vi "USRP Dummy DMA (Host).vi"() -> ()   [LabVIEW 2016]
uses:
  <vilib>/userdefined/High Color/nirio_resource_hc.ctl
  <vilib>/FPGAPlugInAG/USRP 294xR; 295xR 200 MSps/niLvFpga_Open_USRP 294xR; 295xR 200 MSps.vi
  <vilib>/rvi/interface/common/dynamic/niFpgaDynamicAddResources.vi
  <vilib>/Utility/error.llb/Error Cluster From Error Code.vi
  <vilib>/rvi/errors/niLvFpgaAdjustHostInterfaceError.vi
  <vilib>/rvi/interface/common/niFpgaWaitOnOcc.vi
  <vilib>/FPGAPlugInAG/Dynamic/niLvFpga_Close_Dynamic.vi
  <vilib>/rvi/interface/nirviOpenFPGA/nirviOpenFPGA.xnode
  FPGA Bitfiles/USRP-RIO-Streami_DummyDMA_USRPDummy(FPGA)_-Xglc-1l0hs.lvbitx
  <vilib>/rvi/interface/nirviReadWriteControl/nirviReadWriteControl.xnode
  <vilib>/rvi/interface/nirviMethod/nirviMethod.xnode
  <vilib>/rvi/interface/nirviCloseFPGA/nirviCloseFPGA.xnode
  <vilib>/rvi/errors/niLvFpgaMergeErrorWithErrorCode.vi
  <vilib>/rvi/interface/Simulation/niFpgaSimulationCallBeginRW.vi
  <instrlib>/niUsrpRio/Config/v1/Host/niUsrpRio Config v1 Host.lvlib
  NiFpgaLv.dll
  <instrlib>/_niInstr/Basic Elements/v1/FPGA/niInstr Basic Elements v1 FPGA.lvlib
  <vilib>/FPGAPlugInAG/Dynamic/niLvFpga_StopFifo_Dynamic.vi
  <vilib>/FPGAPlugInAG/Dynamic/niLvFpga_ConfigureFifo_Dynamic.vi
  <vilib>/FPGAPlugInAG/Dynamic/niLvFpga_StartFifo_Dynamic.vi
  <vilib>/FPGAPlugInAG/Dynamic/niLvFpga_ReadFifo_Dynamic.vi
panel:
  out "FPGA Side FIFO":cluster{u32, u32}(slide) scale=0.0..1.0
  out "Host Side FIFO":cluster{u32, u32}(slide) scale=0.0..4294967295.0
  out "Data Loop":i32
  out "Fetch Loop":i32
  out "Control Loop":i32
  out "Host Transfer Count":u64
  in  "Number of Samples":u64=1024
  out "FPGA Transfer Count":u64
  in  "Send Data?":bool
  in  "stop":bool
  out "Elements Remaining":u32
  out "Data":u64[](array[numeric]) format="%.0x"
  out "Total Timeouts":u64
  out "Sticky Timeouts?":bool
  in  "Reset Total Timeouts?":bool
  out "Actual Depth":u32
  in  "Requested Depth":u32=1048576
  out "error out":errorcluster
  in  "error in (no error)":errorcluster
  in  "resource name":T1="PXI2Slot18Port1Dev1"
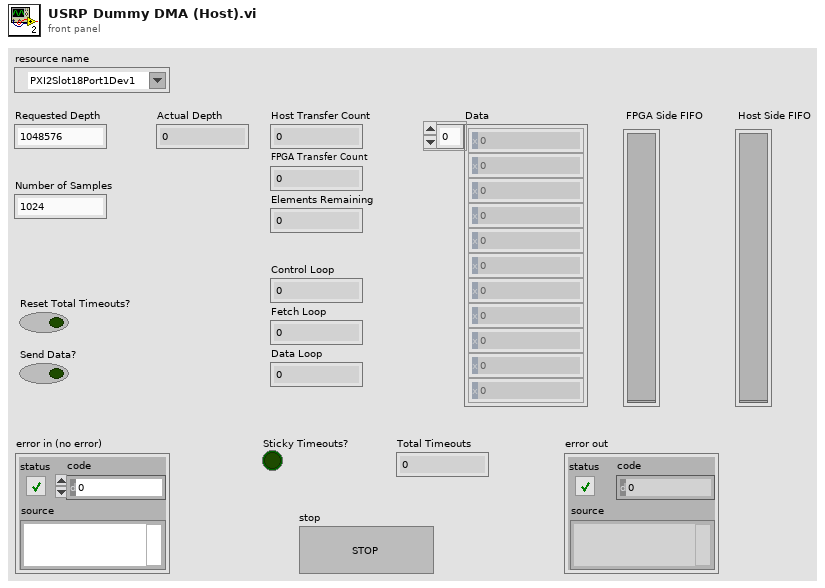
[diagram p1: front panel]
types:
  T1 = typedef "nirio_resource_hc.ctl" = tag
  T2 = typedef "niUsrpRio Config v1 Host.lvlib/niUsrpRio Session.ctl" = cluster{"FPGA Interface":refnum<k20>, "RIO Interface Number":u32, "Data Clock Rate":u32, "FPGA Data Clock Rate":u32, "Global Settings Register Bus":T3, "Radio 0 Settings Register Bus":T3, "Radio 1 Settings Register Bus":T3, "Radio Settings Bus Semaphore":T4, "DB Queues":T5[], "Characterization Data Valid?":bool, "EEPROM Header":T6, "Device Data Header":T7, "EEPROM Characterization Header":T8, "Characterization Data":T9[], "FPGA Current Version":u32, "FPGA Oldest Compatible Version":u32, "Fixed Logic Current Version":u32, "Fixed Logic Oldest Compatible Version":u32, "FPGA Radio Settings Bus Current Version":u32, "FPGA Radio Settings Bus Oldest Compatible Version":u32, "FPGA Board Config Current Version":u32, "FPGA Board Config Oldest Compatible Version":u32, "Daughterboard Clock Rate":u32, "daughterboard configuration session handles":u64[]}
  T3 = typedef "niInstr Register Bus v0 Host.lvlib/Register Bus Session.ctl" = refnum<queue>
  T4 = typedef "Semaphore RefNum" = refnum<k1>
  T5 = typedef "niUsrpRio Config v1 Host.lvlib/DB Queue Reference.ctl" = refnum<queue>
  T6 = typedef "niUsrpRio Config v1 Host.lvlib/EEPROM Header.ctl" = cluster{"Checksum":u32, "Product Code":u16, "Hardware Current Version":u16, "Hardware Oldest Compatible Version":u16, "EEPROM Map Current Version":u16, "EEPROM Map Oldest Compatible Version":u16, "User Password":string, "Pointer to Factory Header":u32, "Pointer to User Header":u32, "Recommended Interval":u16, "Number of Reserved Bytes":i32, "Number of Daughterboards":u8, "Daughterboard IDs":u16[], "Daughterboard Serial Numbers":string[]}
  T7 = typedef "niUsrpRio Config v1 Host.lvlib/EEPROM Device Data Header.ctl" = cluster{"Checksum":u32, "Number of Channels":u8, "Number of Gain Settings":u16[], "Pointer to Characterization Data":u32[], "Number of Reserved Bytes":i32, "Number of Frequencies":u16[]}
  T8 = typedef "niUsrpRio Config v1 Host.lvlib/EEPROM Characterization Header.ctl" = cluster{"Checksum":u32, "Date":timestamp, "Temperature":sgl, "Misc. Info":string, "Pointer to Device Data Header":u32, "Number of Reserved Bytes":i32}
  T9 = typedef "niUsrpRio Config v1 Host.lvlib/Characterization Data.ctl" = cluster{"Gains[dB]":dbl[], "Frequencies [Hz]":dbl[], "IQ Imbalance Table":T10[], "Measured Gains[dB]":dbl[][]}
  T10 = typedef "niUsrpRio Config v1 Host.lvlib/IQ Imbalance.ctl" = cluster{"Gain Imbalance [linear]":dbl, "Phase Imbalance [radians]":dbl, "Offset":cdb}
  T11 = cluster{"Current Amount Used":u32, "Maximum Amount Used":u32}
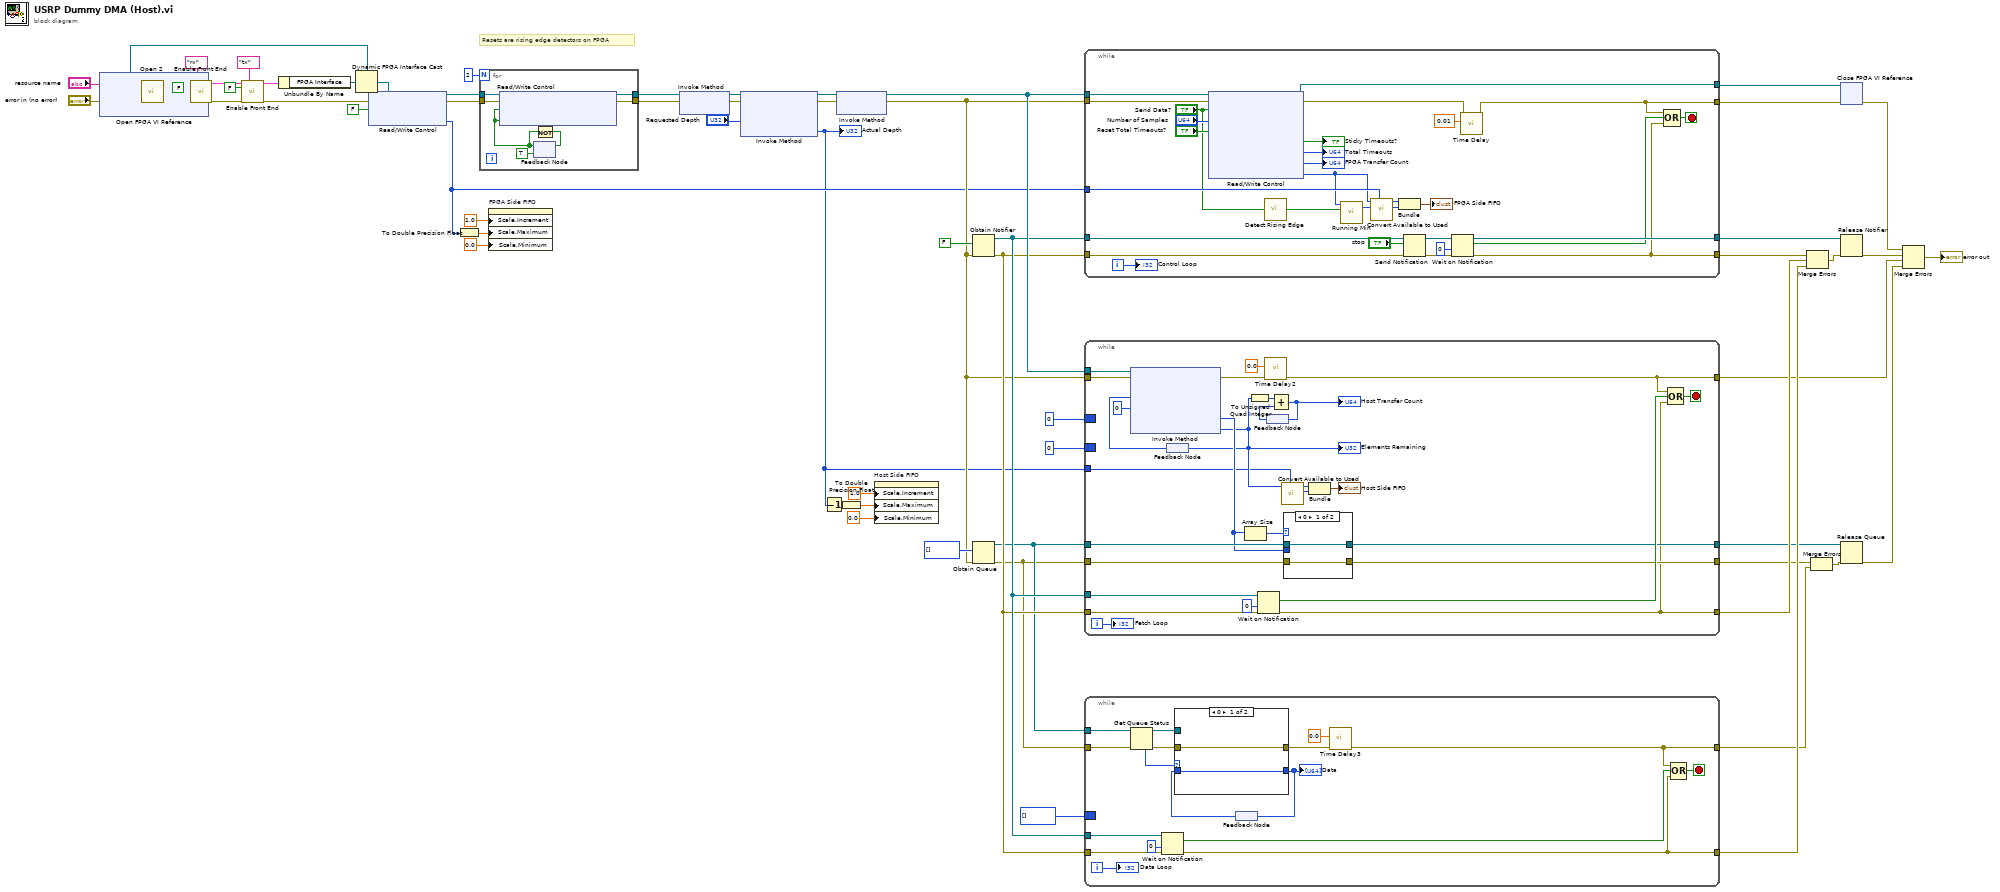
[diagram p0: block diagram]
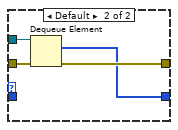
[diagram p2: hidden frame]
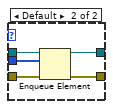
[diagram p3: hidden frame]
diagram:
  # "Resets are rising edge detectors on FPGA"
  n1 = xnode "Open FPGA VI Reference"("error in"="error in (no error)", "resource name"="resource name") -> ("FPGA VI Reference Out"=w42:refnum<k20>, "error out"=w43:errorcluster)
  n2 = call <instrlib>:"Open 2.vi"("fpga ref"=w42, "error in"=w43) -> ("niUsrpRio Session (out)"=w52:T2, "error out"=w57:errorcluster)  [unwired: 12 in]
  n3 = call <instrlib>:"Enable Front End.vi"("niUsrpRio Session"=w52, "scope"="rx", "enable"=FALSE, "error in"=w57) -> ("niUsrpRio Session (out)"=w53:T2, "error out"=w56:errorcluster)  [unwired: 10 in]
  n4 = call <instrlib>:"Enable Front End.vi"("niUsrpRio Session"=w53, "scope"="tx", "enable"=FALSE, "error in"=w56) -> ("niUsrpRio Session (out)"=w49:T2, "error out"=w48:errorcluster)  [unwired: 10 in]
  n5 = Unbundle By Name(w49) -> ("FPGA Interface"=w47:refnum<k20>)
  n6 = Dynamic FPGA Interface Cast(Session In=w42, Type=w47) -> (Session Out=w46:refnum<k20>)
  n7 = xnode "Read/Write Control"("FPGA VI Reference In"=w46, "error in"=w48, "Send Data?"=FALSE ("send data?")) -> ("FPGA VI Reference Out"=w19:refnum<k20>, "error out"=w18:errorcluster, "FPGA FIFO Depth"=w2:u32)
  n8 = To Double Precision Float(number=w2) -> (double precision float=w4:dbl)
  n9 = for {
    N: 2 -> [_]
    tunnel: w19 -> [w70]
    tunnel: w18 -> [w69]
    tunnel: [w68] -> w17
    tunnel: [w67] -> w16
    n10 = feedback #1(TRUE) -> (w65:bool)
    n11 = xnode "Read/Write Control"("FPGA VI Reference In"=w70, "error in"=w69, "Reset Total Timeouts?"=w65, "Reset FPGA Transfer Count?"=w65) -> ("FPGA VI Reference Out"=w68:refnum<k20>, "error out"=w67:errorcluster)
    n12 = Not(x=w65) -> (.not. x?=w64:bool)
    n13 = feedback-in #1(w64) -> ()
  }
  n14 = property on="FPGA Side FIFO" class="Slide (strict)"("Scale.Increment"=1.0 ("Scale.Range:Increment"), "Scale.Maximum"=w4, "Scale.Minimum"=0.0 ("Scale.Range:Minimum")) -> ()  [unwired: 2 in, 2 out]
  n15 = xnode "Invoke Method"("FPGA VI Reference In"=w17, "error in"=w16) -> ("FPGA VI Reference Out"=w63:refnum<k20>, "error out"=w62:errorcluster)
  n16 = xnode "Invoke Method"("FPGA VI Reference In"=w63, "error in"=w62, "Requested Depth"="Requested Depth") -> ("FPGA VI Reference Out"=w59:refnum<k20>, "error out"=w60:errorcluster, "Actual Depth"=w1:u32)
  "Actual Depth" <- w1
  n17 = Decrement(x=w1) -> (x-1=w9:u32)
  n18 = xnode "Invoke Method"("FPGA VI Reference In"=w59, "error in"=w60) -> ("FPGA VI Reference Out"=w41:refnum<k20>, "error out"=w3:errorcluster)
  n19 = To Double Precision Float(number=w9) -> (double precision float=w8:dbl)
  n20 = property on="Host Side FIFO" class="Slide (strict)"("Scale.Increment"=1.0 ("Data Entry Limits:Increment"), "Scale.Maximum"=w8, "Scale.Minimum"=0.0 ("Data Entry Limits:Minimum")) -> ()  [unwired: 2 in, 2 out]
  n21 = Obtain Notifier(notification data type=FALSE, error in (no error)=w3) -> (notifier out=w31:refnum<notifier>, error out=w30:errorcluster)  [unwired: 2 in, 1 out]
  n22 = Obtain Queue(element data type=u64[] [] ("Data"), error in (no error)=w3) -> (queue out=w23:refnum<queue>, error out=w22:errorcluster)  [unwired: 3 in, 1 out]
  n23 = while {
    tunnel: w41 -> [w100]
    tunnel: w3 -> [w99]
    tunnel: w31 -> [w95]
    tunnel: w30 -> [w94]
    tunnel: [w89] -> w37
    tunnel: [w79] -> w36
    tunnel: [w81] -> w14
    tunnel: [w80] -> w13
    tunnel: w2 -> [w78]
    i -> [w86]
    stop <- w88 stop-if-true
    n24 = xnode "Read/Write Control"("FPGA VI Reference In"=w100, "error in"=w99, "Send Data?"="Send Data?", "Number of Samples"="Number of Samples", "Reset Total Timeouts?"="Reset Total Timeouts?") -> ("FPGA VI Reference Out"=w80:refnum<k20>, "error out"=w97:errorcluster, "Sticky Timeout?"=→"Sticky Timeouts?":bool, "Total Timeouts"=→"Total Timeouts":u64, "FPGA Transfer Count"=→"FPGA Transfer Count":u64, "Space Available"=w73:u32)
    n25 = call <instrlib>:"Detect Rising Edge.vi"("signal"="Send Data?") -> ("edge detected"=w71:bool)  [unwired: 14 in]
    n26 = call "Running Min.vi"("Reset"=w71, "Next Value"=w73) -> ("Running Min"=w74:u32)  [unwired: 5 in]
    n27 = call "Convert Available to Used.vi"("Size"=w78, "Minimum Amount Available"=w74, "Current Amount Available"=w73) -> ("Maximum Amount Used"=w76:u32, "Current Amount Used"=w77:u32)  [unwired: 5 in]
    n28 = Bundle("Current Amount Used"=w77, "Maximum Amount Used"=w76) -> (→"FPGA Side FIFO":T11)  [unwired: 1 in]
    n29 = Send Notification(notification="stop", notifier=w95, error in (no error)=w94) -> (notifier out=w91:refnum<notifier>, error out=w90:errorcluster)
    n30 = Wait on Notification(notifier=w91, timeout in ms (-1)=0, error in (no error)=w90) -> (notifier out=w89:refnum<notifier>, notification=w87:bool, error out=w79:errorcluster)  [unwired: 1 in, 1 out]
    n31 = call "Time Delay"("error in (no error)"=w97, "Delay Time (s)"=0.01) -> ("error out"=w81:errorcluster)  [unwired: 9 in]
    n32 = Compound Arithmetic op=OR(w81, w87, w79) -> (w88:bool)
    "Control Loop" <- w86
  }
  n33 = while {
    tunnel: [w121] -> w15
    tunnel: w41 -> [w126]
    tunnel: w3 -> [w125]
    border: u64 0 -> [_]
    border: u32 0 ("Elements Remaining") -> [_]
    tunnel: w31 -> [w117]
    tunnel: w30 -> [w116]
    tunnel: [w106] -> w34
    tunnel: [w112] -> w27
    tunnel: w23 -> [w113]
    tunnel: w22 -> [w111]
    tunnel: [w110] -> w26
    tunnel: w1 -> [w101]
    i -> [w114]
    stop <- w119 stop-if-true
    n34 = feedback #2() -> (w123:u32)
    n35 = xnode "Invoke Method"("FPGA VI Reference In"=w126, "error in"=w125, "Number of Elements"=w123, "Timeout (ms)"=0) -> ("error out"=w109:errorcluster, "Data"=w107:u64[], "Elements Remaining"=w105:u32)  [unwired: 1 out]
    "Elements Remaining" <- w105
    n36 = feedback-in #2(w105) -> ()
    n37 = Array Size(array=w107) -> (size(s)=w108:i32)
    n38 = To Unsigned Quad Integer(1:w105) -> (0:w128:u64)
    n39 = Wait on Notification(notifier=w117, timeout in ms (-1)=0, error in (no error)=w116) -> (notification=w115:bool, error out=w106:errorcluster)  [unwired: 1 in, 2 out]
    n40 = call "Time Delay2"("error in (no error)"=w109, "Delay Time (s)"=0.0) -> ("error out"=w121:errorcluster)  [unwired: 9 in]
    n41 = feedback #3() -> (w127:u64)
    n42 = Add(x=w128, y=w127) -> (x+y=w122:u64)
    "Host Transfer Count" <- w122
    n43 = feedback-in #3(w122) -> ()
    n44 = call "Convert Available to Used.vi"("Size"=w101, "Current Amount Available"=w105) -> ("Maximum Amount Used"=w103:u32, "Current Amount Used"=w104:u32)  [unwired: 6 in]
    n45 = case shown="0" w108 {
      tunnel: w113 -> [w130 w135]
      tunnel: [w130 w134] -> w112
      tunnel: w111 -> [w129 w133]
      tunnel: [w129 w132] -> w110
      tunnel: w107 -> [_ w131]
      frame 0 {
      }
      frame Default {
        n46 = Enqueue Element(queue=w135, element=w131, error in (no error)=w133) -> (queue out=w134:refnum<queue>, error out=w132:errorcluster)  [unwired: 1 in, 1 out]
      }
    }
    n47 = Bundle("Current Amount Used"=w104, "Maximum Amount Used"=w103) -> (→"Host Side FIFO":T11)  [unwired: 1 in]
    n48 = Compound Arithmetic op=OR(w121, w115, w106) -> (w119:bool)
    "Fetch Loop" <- w114
  }
  n49 = while {
    tunnel: w31 -> [w150]
    tunnel: w30 -> [w149]
    tunnel: [w136] -> w29
    tunnel: w23 -> [w147]
    tunnel: w22 -> [w146]
    tunnel: [w138] -> w21
    border: u64[] [] -> [_]
    i -> [w152]
    stop <- w140 stop-if-true
    n50 = Get Queue Status(queue=w147, error in (no error)=w146) -> (queue out=w144:refnum<queue>, error out=w145:errorcluster, # elements in queue=w141:i32)  [unwired: 1 in, 5 out]
    n51 = Wait on Notification(notifier=w150, timeout in ms (-1)=0, error in (no error)=w149) -> (notification=w148:bool, error out=w136:errorcluster)  [unwired: 1 in, 2 out]
    n52 = feedback #4() -> (w143:u64[])
    n53 = case shown="0" w141 {
      tunnel: [w154 w158] -> w139
      tunnel: [w153 w155] -> w142
      tunnel: w145 -> [w154 w157]
      tunnel: w144 -> [_ w156]
      tunnel: w143 -> [w153 _]
      frame 0 {
      }
      frame Default {
        n54 = Dequeue Element(queue=w156, error in (no error)=w157) -> (element=w155:u64[], error out=w158:errorcluster)  [unwired: 1 in, 2 out]
      }
    }
    "Data" <- w142
    n55 = feedback-in #4(w142) -> ()
    n56 = call "Time Delay3"("error in (no error)"=w139, "Delay Time (s)"=0.0) -> ("error out"=w138:errorcluster)  [unwired: 9 in]
    n57 = Compound Arithmetic op=OR(w138, w148, w136) -> (w140:bool)
    "Data Loop" <- w152
  }
  n58 = Merge Errors(w36, w34, w29) -> (w35:errorcluster)
  n59 = Merge Errors(w26, w21) -> (w25:errorcluster)
  n60 = xnode "Close FPGA VI Reference"("FPGA VI Reference In"=w13, "error in"=w14) -> ("error out"=w5:errorcluster)
  n61 = Release Notifier(notifier=w37, error in (no error)=w35) -> (error out=w33:errorcluster)  [unwired: 1 in, 2 out]
  n62 = Release Queue(queue=w27, error in (no error)=w25) -> (error out=w24:errorcluster)  [unwired: 1 in, 2 out]
  n63 = Merge Errors(w5, w33, w15, w24) -> (→"error out":errorcluster)
